vi "Shape to Scan.vi"(0 "X center":dbl, 1 "X size":dbl=10.0, 2 "Ramp down ratio":dbl(slide)=0.1 scale=0.0..1.0, 3 "Y center":dbl, 4 "Y size":dbl=10.0, 5 "X resolution":u32=1024, 8 "Y resolution":u32=768) -> (6 "X scan array":dbl[](graph), 7 "XY scan array":dbl[][](graph), 9 "Y scan array":dbl[](graph))   [LabVIEW 2012]
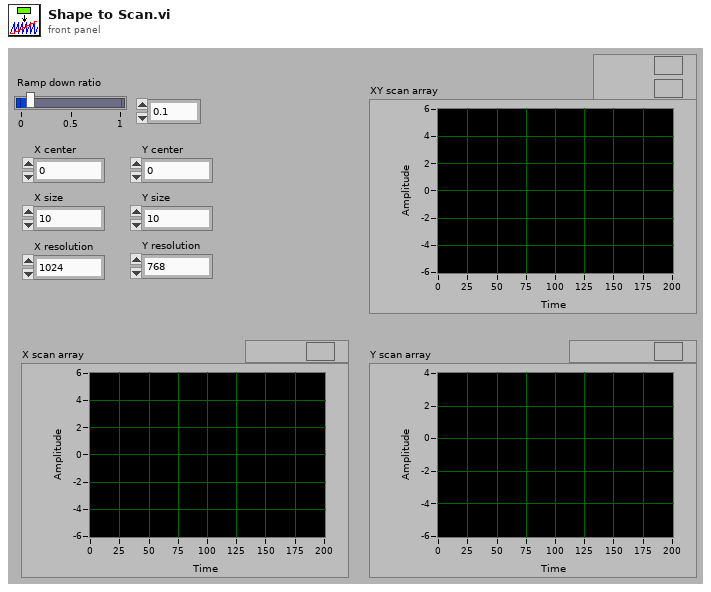
[diagram p1: front panel]
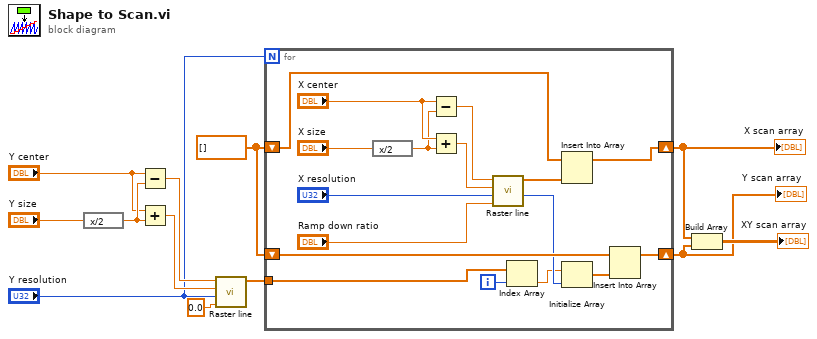
[diagram p0: block diagram]
diagram:
  w1 = dbl[] []
  n1 = expression code="x/2"("Y size") -> (w12:dbl)
  n2 = Subtract(x="Y center", y=w12) -> (x-y=w9:dbl)
  n3 = Add(x="Y center", y=w12) -> (x+y=w8:dbl)
  n4 = call "Raster line.vi"("Ramp down ratio"=0.0, "Points"="Y resolution", "End"=w8, "Start"=w9) -> ("Scan Pattern"=w5:dbl[])  [unwired: 1 in, 6 out]
  n5 = for {
    N: "Y resolution" -> [_]
    shift-right: [w21] -> w3
    shift-left: w1 -> [w20]
    tunnel: w5 -> [w16]
    shift-right: [w19] -> w2
    shift-left: w1 -> [w18]
    i -> [w15]
    n6 = expression code="x/2"("X size") -> (w27:dbl)
    n7 = Subtract(x="X center", y=w27) -> (x-y=w25:dbl)
    n8 = Add(x="X center", y=w27) -> (x+y=w26:dbl)
    n9 = call "Raster line.vi"("Ramp down ratio"="Ramp down ratio", "Points"="X resolution", "End"=w26, "Start"=w25) -> ("Total points"=w17:u32, "Scan Pattern"=w22:dbl[])  [unwired: 1 in, 5 out]
    n10 = Index Array(array=w16, index=w15) -> (element=w14:dbl)
    n11 = Insert Into Array(array=w20, new element=w22) -> (w21:dbl[])  [unwired: 1 in]
    n12 = Initialize Array(w14, w17) -> (w13:dbl[])
    n13 = Insert Into Array(array=w18, new element=w13) -> (w19:dbl[])  [unwired: 1 in]
  }
  "X scan array" <- w3
  "Y scan array" <- w2
  n14 = Build Array(w3, w2) -> (→"XY scan array":dbl[][])
